vi "scroll bar state.vi"(8 "error in (no error)":errorcluster, 10 "Horizontal Scrollbar Visibility":T1(ring), 11 "Pane ref in":refnum<vi>) -> (0 "error out":errorcluster)   [LabVIEW 2015]
panel:
  out "Pane ref out":refnum<vi>
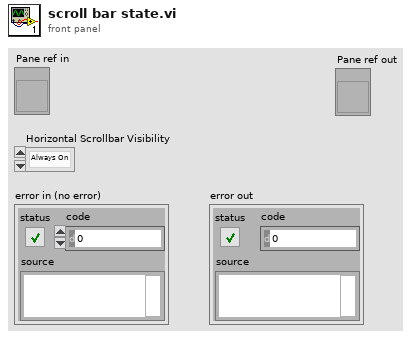
[diagram p1: front panel]
types:
  T1 = enum16{"Always On", "Always Off", "Off While Running"}
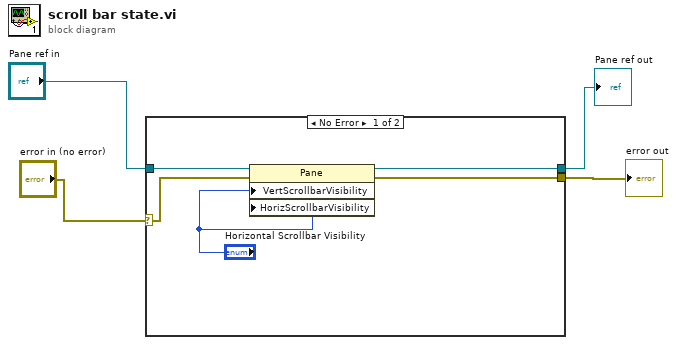
[diagram p0: block diagram]
diagram:
  n1 = case shown="No Error" "error in (no error)" {
    selector: "error in (no error)" -> [w5 w10]
    tunnel: [w9 w10] -> w4
    tunnel: "Pane ref in" -> [w8 w11]
    tunnel: [w7 w11] -> w2
    frame No Error {
      n2 = property on="Property Node" class="Pane"(reference=w8, error in=w5, "VertScrollbarVisibility"="Horizontal Scrollbar Visibility", "HorizScrollbarVisibility"="Horizontal Scrollbar Visibility") -> (reference out=w7:refnum<vi>, error out=w9:errorcluster)
    }
    frame Error {
    }
  }
  "error out" <- w4
  "Pane ref out" <- w2
